vi "Find_first_inactive.vi"(10 "Trial sequence":cluster{"Sequence name":string, "Active":bool}[](array[cluster])) -> (2 "First inactive":i32)   [LabVIEW 2016]
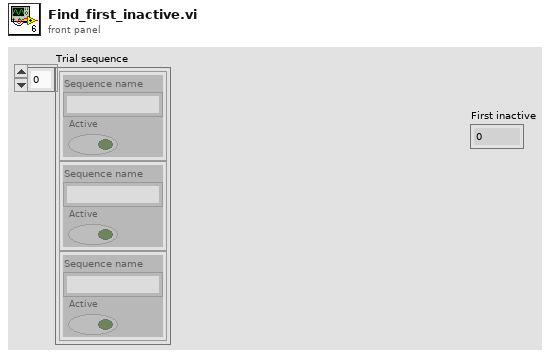
[diagram p1: front panel]
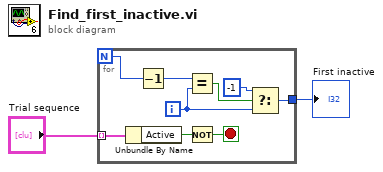
[diagram p0: block diagram]
diagram:
  n1 = for {
    N -> [w8]
    tunnel: "Trial sequence" -> [w11] mode=indexing
    tunnel: [w4] -> w2
    i -> [w5]
    stop <- w9 stop-if-true
    n2 = Unbundle By Name(w11) -> ("Active"=w10:bool)
    n3 = Decrement(x=w8) -> (x-1=w7:i32)
    n4 = Equal?(x=w7, y=w5) -> (x = y?=w6:bool)
    n5 = Not(x=w10) -> (.not. x?=w9:bool)
    n6 = Select(t=-1, s=w6, f=w5) -> (s? t:f=w4:i32)
  }
  "First inactive" <- w2
